vi "Format.vi"(8 "Error in (no error)":errorcluster, 10 "Log in":T1 {"Priority" items=["EMERGENCY", "ALERT", "CRITICAL", "ERROR", "WARNING", "NOTICE", "INFO", "DEBUG"]}, 11 "LogFormatterSimple in":refnum<class "LogFormatterSimple.lvclass">) -> (0 "Error out":errorcluster, 2 "Log formatted":string, 3 "LogFormatterSimple out":refnum<class "LogFormatterSimple.lvclass">)   [LabVIEW 2011, in "LogFormatterSimple.lvclass"]
uses:
  LogFormatterSimple.lvclass
  Log/LogCluster.ctl
  Log/PrioritiesRing.ctl
  LogFormatterSimple.lvclass/LogFormatterSimple.ctl
  Log/Log.lvclass
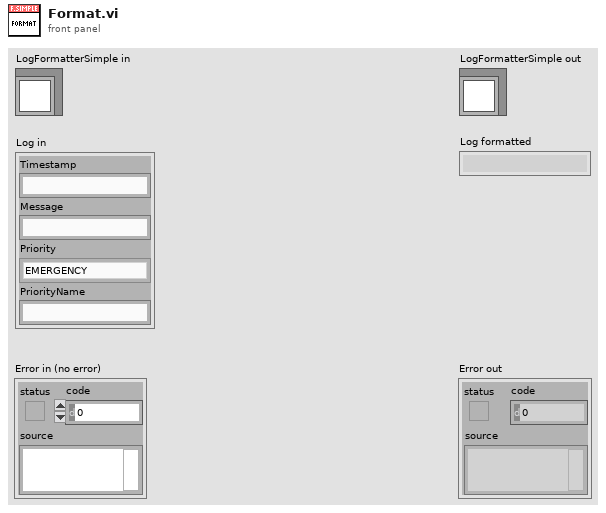
[diagram p1: front panel]
types:
  T1 = typedef "Log.lvclass/LogCluster.ctl" = cluster{"Timestamp":string, "Message":string, "Priority":T2, "PriorityName":string}
  T2 = typedef "Log.lvclass/PrioritiesRing.ctl" = u32
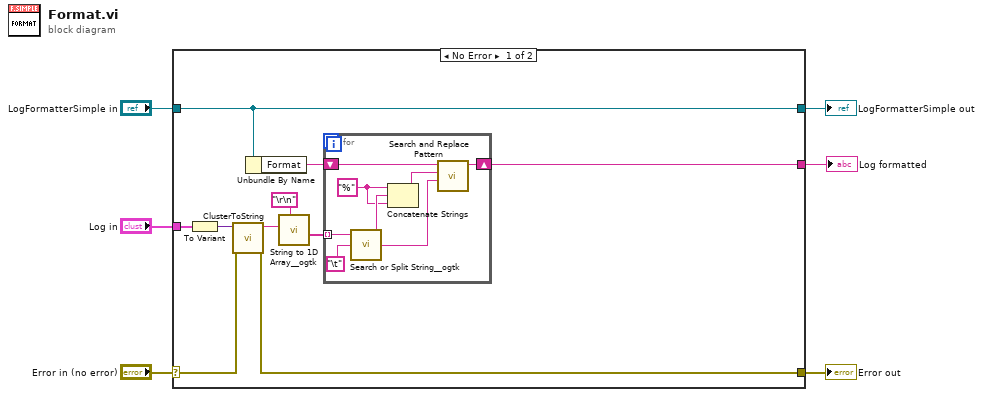
[diagram p0: block diagram]
diagram:
  n1 = case shown="No Error" "Error in (no error)" {
    selector: "Error in (no error)" -> [w14 w26]
    tunnel: [w13 w26] -> w5
    tunnel: [w16 w25] -> w3
    tunnel: "LogFormatterSimple in" -> [w16 w25]
    tunnel: "Log in" -> [w15 _]
    tunnel: [w8 _] -> w1
    frame No Error {
      n2 = To Variant(anything=w15) -> (Variant=w7:variant)
      n3 = call "ClusterToString.vi"("Error in (no error)"=w14, "Cluster"=w7) -> ("Error out"=w13:errorcluster, "String out"=w12:string)  [unwired: 8 in]
      n4 = Unbundle By Name(w16) -> ("Format"=w9:string)
      n5 = call <userlib>:"String to 1D Array__ogtk.vi"("delimiter (Tab)"="\r\n", "string"=w12) -> ("Array of Strings"=w10:string[])  [unwired: 9 in]
      n6 = for {
        tunnel: w10 -> [w24] mode=indexing
        shift-right: [w17] -> w8
        shift-left: w9 -> [w22]
        w20 = "%" ("string")
        n7 = call <userlib>:"Search or Split String__ogtk.vi"("search string/char (-)"="\t", "string"=w24) -> ("substring after match"=w18:string, "substring before match"=w21:string)  [unwired: 1 in, 1 out]
        n8 = Concatenate Strings(w20, w21, w20) -> (w19:string)
        n9 = call <vilib>:"Search and Replace Pattern.vi"("string"=w22, "regular expression (\"\")"=w19, "replace string (\"\")"=w18) -> ("result string"=w17:string)  [unwired: 2 in, 1 out]
      }
    }
    frame Error {
    }
  }
  "Error out" <- w5
  "LogFormatterSimple out" <- w3
  "Log formatted" <- w1
